vi "close_roi_file.vi"(8 "error in (no error)":errorcluster, 11 "Camera in":refnum<class "Camera.lvclass">) -> (0 "error out":errorcluster, 3 "Camera out":refnum<class "Camera.lvclass">)   [LabVIEW 2013, in "Camera.lvclass"]
uses:
  Camera.lvclass
panel:
  out "path":path
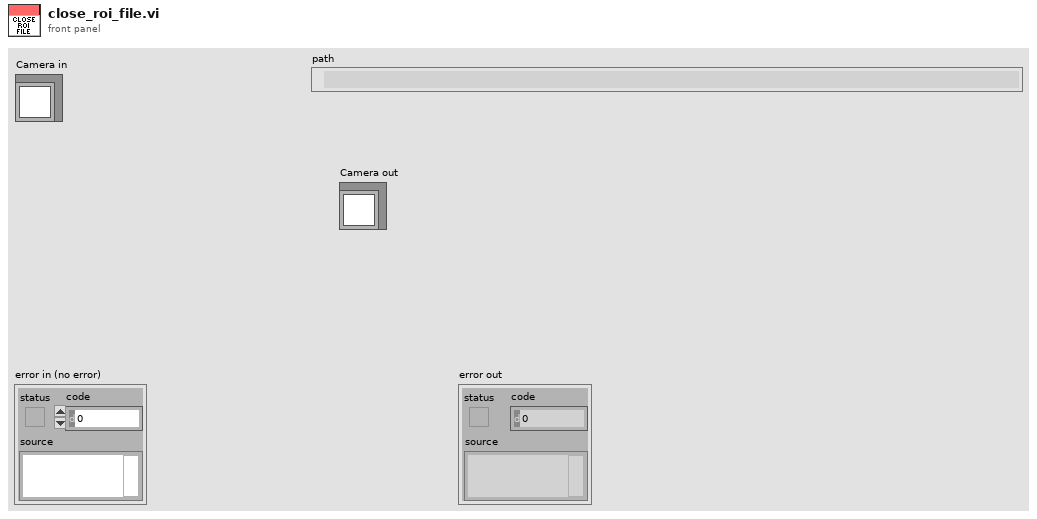
[diagram p1: front panel]
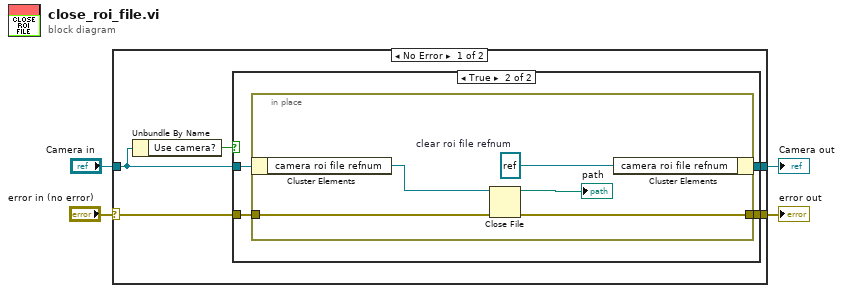
[diagram p0: block diagram]
diagram:
  n1 = case shown="No Error" "error in (no error)" {
    selector: "error in (no error)" -> [w5 w22]
    tunnel: [w6 w22] -> w3
    tunnel: [w7 w21] -> w1
    tunnel: "Camera in" -> [w9 w21]
    frame No Error {
      n2 = Unbundle By Name(w9) -> ("Use camera?"=w8:bool)
      n3 = case shown="True" w8 {
        tunnel: [w10 w15] -> w6
        tunnel: [w11 w14] -> w7
        tunnel: w9 -> [w11 w13]
        tunnel: w5 -> [w10 w12]
        frame False {
        }
        frame True {
          n4 = in-place {
            in-place-border: [w20] -> w15
            in-place-border: w12 -> [w18]
            w17 = refnum<file> refnum  # clear roi file refnum
            n5 = in-place-cluster #1(w13) -> ("camera roi file refnum"=w19:refnum<file>)
            n6 = Close File(refnum=w19, error in=w18) -> (path=→"path":path, error out=w20:errorcluster)
            n7 = in-place-cluster #1("camera roi file refnum"=w17) -> (w14:refnum<class "Camera.lvclass">)
          }
        }
      }
    }
    frame Error {
    }
  }
  "error out" <- w3
  "Camera out" <- w1
